vi "Ctor.vi"(8 "error in (no error)":errorcluster) -> (0 "error out":errorcluster, 3 "HAL Editor out":refnum<class "HAL Editor.lvclass">)   [LabVIEW 2020, in "HAL Config.lvlib" / "HAL Editor.lvclass"]
uses:
  HAL Editor.lvclass
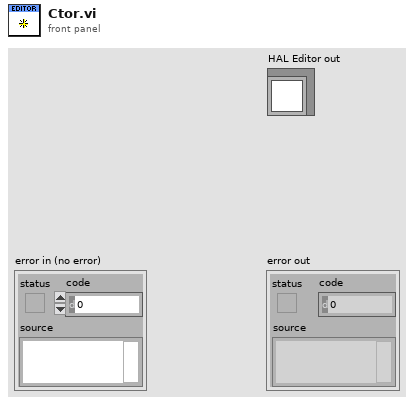
[diagram p1: front panel]
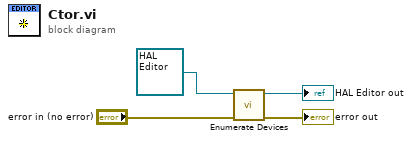
[diagram p0: block diagram]
diagram:
  n1 = call "Enumerate Devices.vi"("error in (no error)"="error in (no error)", "HAL Editor in"=refnum<class "HAL Editor.lvclass"> refnum) -> ("error out"=→"error out":errorcluster, "HAL Editor out"=→"HAL Editor out":refnum<class "HAL Editor.lvclass">)  [unwired: 8 in]
